vi "xiLIB - SaveToINI.vi"(6 "IniPath":path, 8 "error in (no error)":errorcluster, 9 "PRM[] to Save":T1[](array[typedef]), 11 "xiCam":refnum<k24>) -> (0 "error out":errorcluster, 3 "xiCam Out":refnum<k24>)   [LabVIEW 2013]
doc: "Dialog based parameter save function."
uses:
  xiCam/PRM/PRM/PRM_v2.ctl
  C:/Projects/Cameras3.x/xiLib/xiLIB_64bit/xiLIB/xiCamLib/API/x64/xiApi.NETX64.dll
  xiLIB_64bit/xiLIB/xiCamLib/API/x64/xiApi.NETX64.dll
  <vilib>/Utility/config.llb/Write Key (I32).vi
  <vilib>/Utility/config.llb/Write Key (Double).vi
  <vilib>/Utility/config.llb/Write Key (String).vi
  <vilib>/Utility/config.llb/NI_LVConfig.lvlib
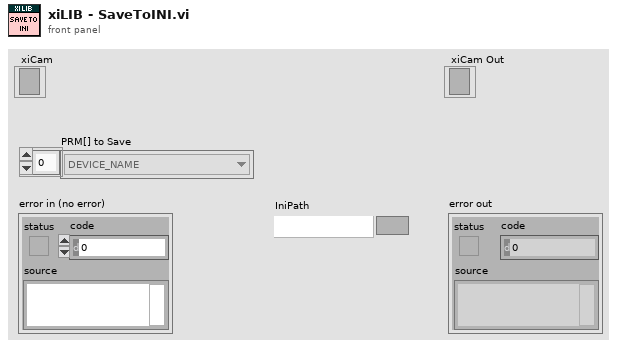
[diagram p1: front panel]
types:
  T1 = typedef "PRM_v2.ctl" = enum16{"ACQ_BUFFER_SIZE", "ACQ_FRAME_BURST_COUNT", "ACQ_TIMING_MODE", "ACQ_TRANSPORT_BUFFER_SIZE", "AE_MAX_LIMIT", "AEAG", "AEAG_LEVEL", "API_VERSION", "AG_MAX_LIMIT", "APPLY_CMS", "AUTO_BANDWIDTH_CALCULATION", "AUTO_WB", "AVAILABLE_BANDWIDTH", "AVAILABLE_BANDWIDTH_MAX", "AVAILABLE_BANDWIDTH_MIN", "BPC", "BUFFER_POLICY", "BUFFERS_QUEUE_SIZE", "CC_MATRIX_00", "CC_MATRIX_01", "CC_MATRIX_02", "CC_MATRIX_03", "CC_MATRIX_10", "CC_MATRIX_11", "CC_MATRIX_12", "CC_MATRIX_13", "CC_MATRIX_20", "CC_MATRIX_21", "CC_MATRIX_22", "CC_MATRIX_23", "CC_MATRIX_30", "CC_MATRIX_31", "CC_MATRIX_32", "CC_MATRIX_33", "CHIP_TEMP", "CMS", "COLOR_FILTER_ARRAY", "COOLING", "DEBOUNCE_EN", "DEBOUNCE_POL", "DEBOUNCE_T0", "DEBOUNCE_T1", "DEBUG_LEVEL", "DEFAULT_CC_MATRIX", "DEVICE_INSTANCE_PATH", "DEVICE_MODEL_ID", "DEVICE_NAME", "DEVICE_SN", "DEVICE_TYPE", "DEVICE_USER_ID", "DOWNSAMPLING", "DOWNSAMPLING_MAX", "DOWNSAMPLING_MIN", "DOWNSAMPLING_TYPE", "DRV_VERSION", "EXP_PRIORITY", "EXPOSURE", "EXPOSURE_DIRECT_UPDATE", "EXPOSURE_MAX", "EXPOSURE_MIN", "FFS_FILE_NAME", "FPGA1_VERSION", "FRAMERATE", "FRAMERATE_MAX", "FRAMERATE_MIN", "FREE_FFS_SIZE", "GAIN", "GAIN_DIRECT_UPDATE", "GAIN_MAX", "GAIN_MIN", "GAMMAC", "GAMMAY", "GPI_LEVEL", "GPI_MODE", "GPI_SELECTOR", "GPI_SELECTOR_MAX", "GPI_SELECTOR_MIN", "GPO_MODE", "GPO_SELECTOR", "GPO_SELECTOR_MAX", "GPO_SELECTOR_MIN", "HDR", "HDR_T1", "HDR_T2", "HEIGHT", "HEIGHT_MAX", "HEIGHT_MIN", "HOUSE_TEMP", "IMAGE_DATA_FORMAT", "IMAGE_IS_COLOR", "INPUT_CMS_PROFILE", "IS_COOLED", "IS_DEVICE_EXIST", "KNEEPOINT1", "KNEEPOINT2", "LED_MODE", "LED_SELECTOR", "LED_SELECTOR_MAX", "LED_SELECTOR_MIN", "LIMIT_BANDWIDTH", "LIMIT_BANDWIDTH_MAX", "LIMIT_BANDWIDTH_MIN", "LUT_EN", "LUT_INDEX", "LUT_INDEX_MAX", "LUT_INDEX_MIN", "LUT_VALUE", "LUT_VALUE_MAX", "LUT_VALUE_MIN", "MANUAL_WB", "MCU1_VERSION", "MCU2_VERSION", "OFFSET_X", "OFFSET_X_MAX", "OFFSET_X_MIN", "OFFSET_Y", "OFFSET_Y_MAX", "OFFSET_Y_MIN", "OUTPUT_CMS_PROFILE", "OUTPUT_DATA_BIT_DEPTH", "OUTPUT_DATA_PACKING", "READ_FILE_FFS", "RECENT_FRAME", "SENSOR_DATA_BIT_DEPTH", "SENSOR_MODE", "SENSOR_TAPS", "SHARPNESS", "SHUTTER_TYPE", "TARGET_TEMP", "TRG_DELAY", "TRG_SELECTOR", "TRG_SOFTWARE", "TRG_SOURCE", "USED_FFS_SIZE", "WB_KB", "WB_KG", "WB_KR", "WIDTH", "WIDTH_MAX", "WIDTH_MIN", "WRITE_FILE_FFS", "ACQ_BUFFER_SIZE_UNIT", "ACQ_TRANSPORT_BUFFER_COMMIT", "AEAG_ROI_HEIGHT", "AEAG_ROI_OFFSET_X", "AEAG_ROU_OFFSET_Y", "AEAG_ROI_WIDTH", "API_CONTEXT_LIST", "BINNING_HORIZONTAL", "BINNING_PATTERN", "BINNING_SELECTOR", "BINNING_VERTICAL", "COLUMN_FPN_CORRECTION", "COUNTER_SELECTOR", "COUNTER_VALUE", "DECIMATION_HORIZONTAL", "DECIMATION_PATTERN", "DECIMATION_SELECTOR", "DECIMATION_VERTICAL", "DEVICE_ID", "DEVICE_LOCATION_PATH", "DEVICE_MANIFEST", "DEVICE_RESET", "DEVICE_SENS_SN", "EXPOSURE_BURST_COUNT", "FFS_ACCESS_KEY", "GAIN_SELECTOR", "HW_REVISION", "IMAGE_BLACK_LEVEL", "IMAGE_DATA_BIT_DEPTH", "IMAGE_DATA_FORMAT_RGB32_ALPHA", "IMAGE_PAYLOAD_SIZE", "LENS_APERTURE_VALUE", "LENS_FEATURE", "LENS_FEATURE_SELECTOR", "LENS_FOCAL_LENGTH", "LENS_FOCUS_DISTANCE", "LENS_FOCUS_MOVE", "LENS_FOCUS_MOVEMENT_VALUE", "LENS_MODE", "OUTPUT_DATA_PACKING_TYPE", "SENSOR_CLOCK_FREQ_HZ", "SENSOR_CLOCK_FREQ_INDEX", "SENSOR_FEATURE_SELECTOR", "SENSOR_FEATURE_VALUE", "SENSOR_OUTPUT_CHANNEL_COUNT", "TRANSPORT_PIXEL_FORMAT", "TS_RST_MODE", "TS_RST_SOURCE"}
  T2 = typedef "NI_LVConfig.lvlib/Config Data RefNum.ctl" = refnum<k1>
  T3 = typedef "xiLIB - PRM_Attribute.ctl" = cluster{"Type":T4, "Method":T5, "Desc.":string, "PRM":T1}
  T4 = typedef "xiLIB - PRM_Type.ctl" = enum16{"Int32", "Float", "String", "DOWNSAMPLING_TYPE", "IMAGE_DATA_FORMAT", "BUFFER_POLICY", "TRG_SOURCE", "GPI", "GPO", "ACQ_TIMING_MODE", "BINNING_PATTERN", "BINNING_SELECTOR", "CMS_MODE", "COUNTER_SELECTOR", "DEBUG_LEVEL", "DECIMATION_PATTERN", "DECIMATION_SELECTOR", "GAIN_SELECTOR_TYPE", "LED_MODE", "LENS_FEATURE_SELECTOR", "LENS_MODE", "OUTPUT_DATA_PACKING_TYPE", "SENSOR_FEATURE_SELECTOR", "SHUTTER_TYPE", "TRG_SELECTOR", "TS_RST_MODE", "TS_RST_SOURCE"}
  T5 = typedef "xiLIB - PRM_Function.ctl" = enum16{"Get / Set", "Get", "Set"}
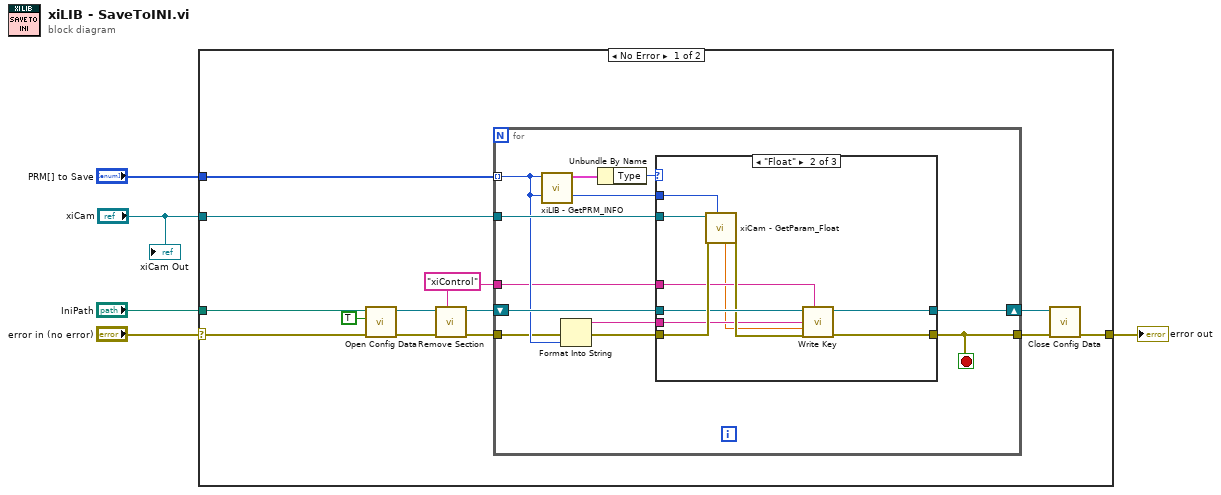
[diagram p0: block diagram]
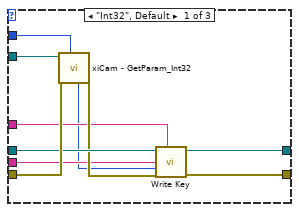
[diagram p2: hidden frame]
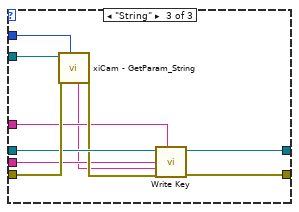
[diagram p3: hidden frame]
diagram:
  n1 = case shown="No Error" "error in (no error)" {
    selector: "error in (no error)" -> [w17 w60]
    tunnel: [w6 w60] -> w4
    tunnel: "IniPath" -> [w18 _]
    tunnel: "PRM[] to Save" -> [w9 _]
    tunnel: "xiCam" -> [w8 _]
    frame No Error {
      w11 = "xiControl" ("section")
      n2 = call <vilib>:"Open Config Data.vi"("error in (no error)"=w17, "create file if necessary (T)"=TRUE, "configuration file path"=w18) -> ("error out"=w15:errorcluster, "refnum"=w14:T2)  [unwired: 6 in, 1 out]
      n3 = call <vilib>:"Remove Section.vi"("section"=w11, "error in (no error)"=w15, "refnum"=w14) -> ("error out"=w12:errorcluster, "refnum out"=w13:T2)  [unwired: 6 in, 1 out]
      n4 = for {
        tunnel: w8 -> [w27]
        tunnel: w9 -> [w25] mode=indexing
        tunnel: w12 -> [w24]
        tunnel: w11 -> [w22]
        shift-right: [w20] -> w10
        shift-left: w13 -> [w26]
        tunnel: [w19] -> w7
        stop <- w19 stop-if-true
        n5 = call "xiLIB - GetPRM_INFO.vi"("PRM"=w25) -> ("PRM_Attributes"=w29:T3)  [unwired: 10 in]
        n6 = Format Into String(error in=w24, w25) -> (resulting string=w21:string, error out=w23:errorcluster)  [unwired: 2 in]
        n7 = Unbundle By Name(w29) -> ("Type"=w28:T4)
        n8 = case shown="\"Float\"" w28 {
          tunnel: w27 -> [w30 w40 w50]
          tunnel: w25 -> [w39 w49 w59]
          tunnel: w23 -> [w38 w48 w58]
          tunnel: w26 -> [w37 w47 w57]
          tunnel: w21 -> [w35 w45 w55]
          tunnel: w22 -> [w34 w44 w54]
          tunnel: [w32 w42 w52] -> w20
          tunnel: [w31 w41 w51] -> w19
          frame "Int32", Default {
            n9 = call "xiCam - GetParam_Int32.vi"("PRM"=w39, "error in (no error)"=w38, "xiCam In"=w30) -> ("error out"=w36:errorcluster, "Int32_Value"=w33:i32)  [unwired: 6 in, 1 out]
            n10 = call-poly <vilib>:"Write Key.vi"("section"=w34, "error in (no error)"=w36, "value"=w33, "key"=w35, "refnum"=w37) -> ("error out"=w31:errorcluster, "refnum out"=w32:T2)  [unwired: 4 in, 1 out]
          }
          frame "Float" {
            n11 = call "xiCam - GetParam_Float.vi"("PRM"=w49, "error in (no error)"=w48, "xiCam In"=w40) -> ("error out"=w46:errorcluster, "Float_Value"=w43:sgl)  [unwired: 6 in, 1 out]
            n12 = call-poly <vilib>:"Write Key.vi"("section"=w44, "error in (no error)"=w46, "value"=w43, "key"=w45, "refnum"=w47) -> ("error out"=w41:errorcluster, "refnum out"=w42:T2)  [unwired: 4 in, 1 out]
          }
          frame "String" {
            n13 = call "xiCam - GetParam_String.vi"("PRM"=w59, "error in (no error)"=w58, "xiCam In"=w50) -> ("error out"=w56:errorcluster, "String_Value"=w53:string)  [unwired: 6 in, 1 out]
            n14 = call-poly <vilib>:"Write Key.vi"("section"=w54, "error in (no error)"=w56, "value"=w53, "key"=w55, "refnum"=w57) -> ("error out"=w51:errorcluster, "refnum out"=w52:T2)  [unwired: 4 in, 1 out]
          }
        }
      }
      n15 = call <vilib>:"Close Config Data.vi"("error in (no error)"=w7, "refnum"=w10) -> ("error out"=w6:errorcluster)  [unwired: 8 in, 1 out]
    }
    frame Error {
    }
  }
  "error out" <- w4
  "xiCam Out" <- "xiCam"
